vi "Move From Output to Export Dir.vi"(0 "NI Build Specification in":refnum<class "SourceDist_LV.lvclass">, 11 "error IO":errorcluster) -> (4 "NI Build Specification out":refnum<class "SourceDist_LV.lvclass">, 15 "error out":errorcluster)   [LabVIEW 2017, in "CL_G3_VIComponentBuilder.lvlib" / "SourceDist_LV.lvclass"]
doc: "Place source distribution files in a new directory named after the build spec name of the source dir. This new directory is placed into the component's export directory."
uses:
  SourceDist_LV.lvclass
  C:/builds/Component BuilderBT/SrcDist/Exports/Exports/Export.lvclass
  C:/builds/Component BuilderBT/SrcDist/Exports/NI Build Specification_LV/NI Build Specification_LV.lvclass
  <vilib>/AppBuilder/AB_API/common/AB_API Build Object Selector.ctl
  Exports/Export.lvclass/Export.ctl
  NI Build Specification_LV/NI Build Specification_LV.lvclass/NI Build Specification_LV.ctl
  Exports/Accessors/Read Component Export Dir.vi
  NI Build Specification_LV/Accessors/Read Export's Build Spec Name.vi
  NI Build Specification_LV/Accessors/Read TargetRef Containting Build Spec.vi
  NI Build Specification_LV/Accessors/Read Project Reference.vi
  Exports/Accessors/Write Built Export's Full Path.vi
  <vilib>/Utility/file.llb/Is Path and Not Empty.vi
  <vilib>/Utility/libraryn.llb/Check if File or Folder Exists.vi
  <vilib>/Utility/error.llb/Error Cluster From Error Code.vi
  <vilib>/AppBuilder/AB_API/Build/NI_AB_API_Build.lvclass
  NI Build Specification_LV/NI Build Specification_LV.lvclass
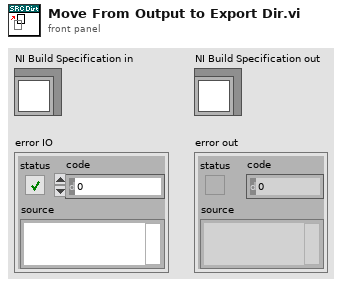
[diagram p1: front panel]
types:
  T1 = typedef "AB_API Build Object Selector.ctl" = enum16{"Source Distribution", "Deployable Source Distribution", "DLL", "EXE", "Packed Library", "Deployable Packed Library", "RT EXE", ".NET Interop Assembly"}
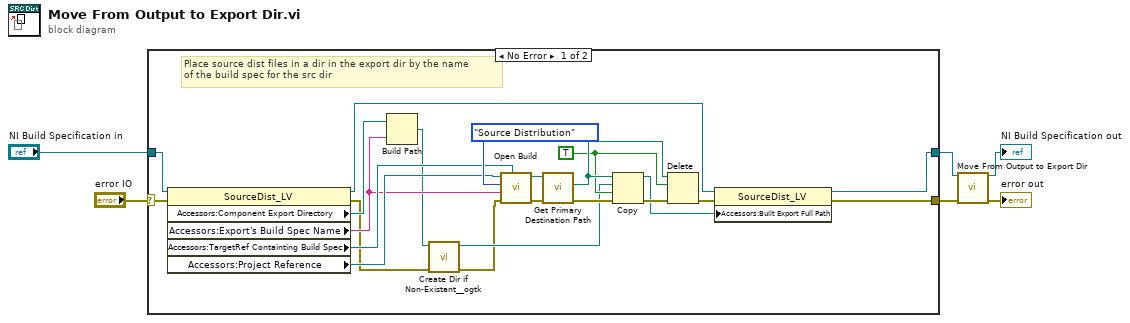
[diagram p0: block diagram]
diagram:
  n1 = case shown="No Error" "error IO" {
    selector: "error IO" -> [w20 w29]
    tunnel: "NI Build Specification in" -> [w21 w30]
    tunnel: [w18 w30] -> w2
    tunnel: [w15 w29] -> w1
    frame No Error {
      w11 = TRUE ("overwrite (F)")
      # "Place source dist files in a dir in the export dir by the name \nof the build spec for the src dir"
      n2 = property class="SourceDist_LV"(reference=w21, error in=w20) -> (reference out=w19:refnum<class "SourceDist_LV.lvclass">, error out=w8:errorcluster, "Accessors:Component Export Directory"=w13:path, "Accessors:Export's Build Spec Name"=w12:string, "Accessors:TargetRef Containting Build Spec"=w23:refnum<vi>, "Accessors:Project Reference"=w26:refnum<vi>)
      n3 = Build Path(base path=w13, name or relative path=w12) -> (appended path=w10:path)
      n4 = call <userlib>:"Create Dir if Non-Existant__ogtk.vi"("error in (no error)"=w8, "Directory Path"=w10) -> ("error out"=w7:errorcluster, "dup Directory Path"=w9:path)  [unwired: 7 in, 1 out]
      n5 = call <vilib>:"Open Build.vi"("TargetItem Refnum"=w23, "error in (no error)"=w7, "Build specification name"=w12, "Build object selector"=AB_API_Build_Object_Selector."Source Distribution", "Project Refnum"=w26) -> ("error out"=w25:errorcluster, "NI_AB_API_Build out"=w28:refnum<class "NI_AB_API_Build.lvclass">)  [unwired: 5 in]
      n6 = call-dynamic "Get Primary Destination Path.vi"("error in (no error)"=w25, "NI_AB_API_Build in"=w28) -> ("error out"=w24:errorcluster, "Primary destination path"=w14:path)  [unwired: 7 in, 1 out]
      n7 = Copy(8:w24, 9:w11, 10:w9, 11:w14) -> (0:w22:errorcluster, 3:w17:path)  [unwired: 1 in, 1 out]
      n8 = Delete(path (use dialog)=w14, entire hierarchy (F)=w11, error in=w22) -> (error out=w16:errorcluster)  [unwired: 2 in, 2 out]
      n9 = property class="SourceDist_LV"(reference=w19, error in=w16, "Accessors:Built Export Full Path"=w17) -> (reference out=w18:refnum<class "SourceDist_LV.lvclass">, error out=w15:errorcluster)
    }
    frame Error {
    }
  }
  n10 = call-parent "Move From Output to Export Dir.vi"("NI Build Specification in"=w2, "error IO"=w1) -> ("NI Build Specification out"=→"NI Build Specification out":refnum<class "SourceDist_LV.lvclass">, "error out"=→"error out":errorcluster)  [unwired: 12 in]
